vi "bmi calculator.vi"() -> ()   [LabVIEW 2019]
panel:
  in  "Tab Control":enum32{"BMI Calculator"}(tab)
  out "Weight Status":string
  out "Your BMI":dbl
  out "Warning!":bool
  in  "stop":bool
  in  "Height (in)":dbl
  in  "Weight (lbs)":dbl
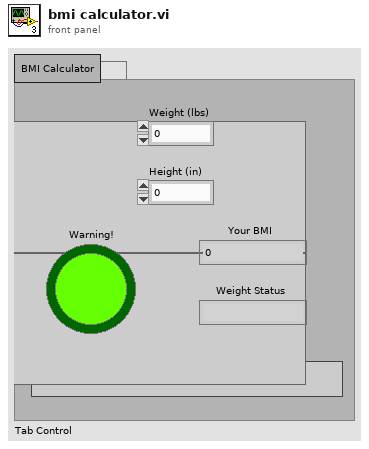
[diagram p1: front panel]
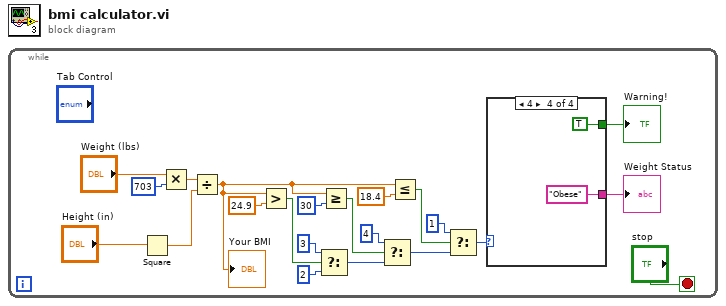
[diagram p0: block diagram]
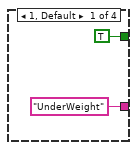
[diagram p2: hidden frame]
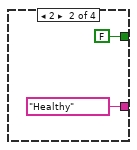
[diagram p3: hidden frame]
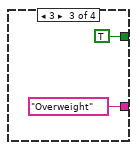
[diagram p4: hidden frame]
diagram:
  n1 = while {
    stop <- "stop" stop-if-true
    n2 = Square(x="Height (in)") -> (x^2=w20:dbl)
    n3 = Multiply(x="Weight (lbs)", y=703) -> (x*y=w18:dbl)
    n4 = Divide(x=w18, y=w20) -> (x/y=w4:dbl)
    "Your BMI" <- w4
    n5 = Greater?(x=w4, y=24.9) -> (0:w11:bool)
    n6 = Select(t=3, s=w11, f=2) -> (s? t:f=w5:i32)
    n7 = Greater Or Equal?(x=w4, y=30) -> (x >= y?=w3:bool)
    n8 = Select(t=4, s=w3, f=w5) -> (s? t:f=w6:i32)
    n9 = Less Or Equal?(x=w4, y=18.4) -> (x <= y?=w8:bool)
    n10 = Select(t=1, s=w8, f=w6) -> (s? t:f=w10:i32)
    n11 = case shown="4" w10 {
      tunnel: ["UnderWeight" "Healthy" "Overweight" "Obese"] -> w17
      tunnel: [TRUE FALSE TRUE TRUE] -> w1
      frame 1, Default {
      }
      frame 2 {
      }
      frame 3 {
      }
      frame 4 {
      }
    }
    "Weight Status" <- w17
    "Warning!" <- w1
  }
